vi "zad4a.vi"   [LabVIEW 2017]
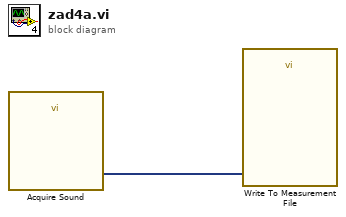
[diagram p0: block diagram]
diagram:
  n1 = call "Acquire Sound"() -> ("Data"=w1:dynamicdata)  [unwired: 18 in, 1 out]
  n2 = call "Write To Measurement File"("Signals"=w1) -> ()  [unwired: 16 in, 3 out]
